vi "Intersect of Line Descriptors.vi"(2 "Line B":T1, 3 "Line A":T1) -> (0 "Intersect":cluster{"X":dbl, "Y":dbl})   [LabVIEW 2012]
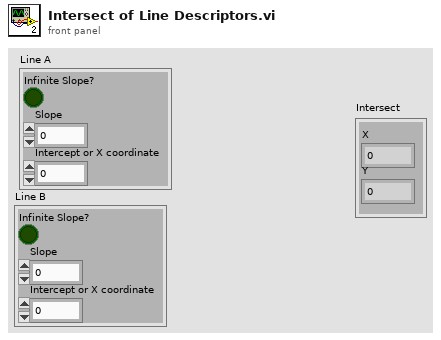
[diagram p1: front panel]
types:
  T1 = cluster{"Infinite Slope?":bool, "Slope":dbl, "Intercept or X coordinate":dbl}
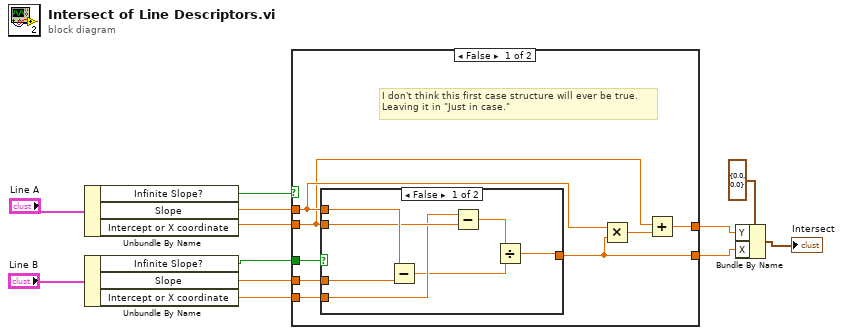
[diagram p0: block diagram]
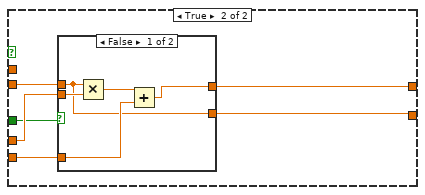
[diagram p3: hidden frame]
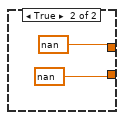
[diagram p4: hidden frame]
diagram:
  n1 = Unbundle By Name("Line A") -> ("Infinite Slope?"=w7:bool, "Slope"=w6:dbl, "Intercept or X coordinate"=w5:dbl)
  n2 = Unbundle By Name("Line B") -> ("Infinite Slope?"=w8:bool, "Slope"=w11:dbl, "Intercept or X coordinate"=w12:dbl)
  n3 = case shown="False" w7 {
    tunnel: w12 -> [w18 w33]
    tunnel: w11 -> [w19 w34]
    tunnel: w8 -> [w20 w30]
    tunnel: w6 -> [w17 _]
    tunnel: w5 -> [w15 w31]
    tunnel: [w14 w29] -> w3
    tunnel: [w13 w32] -> w2
    frame False {
      # "I don't think this first case structure will ever be true.\nLeaving it in \"Just in case.\""
      n4 = case shown="False" w20 {
        tunnel: w17 -> [w27 _]
        tunnel: w15 -> [w25 _]
        tunnel: w19 -> [w26 _]
        tunnel: w18 -> [w24 w28]
        tunnel: [w21 w28] -> w14
        frame False {
          n5 = Subtract(x=w27, y=w26) -> (x-y=w23:dbl)
          n6 = Subtract(x=w24, y=w25) -> (x-y=w22:dbl)
          n7 = Divide(x=w22, y=w23) -> (x/y=w21:dbl)
        }
        frame True {
        }
      }
      n8 = Multiply(x=w17, y=w14) -> (x*y=w16:dbl)
      n9 = Add(x=w15, y=w16) -> (x+y=w13:dbl)
    }
    frame True {
      n10 = case shown="False" w30 {
        tunnel: w34 -> [w39 _]
        tunnel: w33 -> [w37 _]
        tunnel: [w36 nan] -> w32
        tunnel: w31 -> [w35 _]
        tunnel: [w35 nan] -> w29
        frame False {
          n11 = Multiply(x=w35, y=w39) -> (x*y=w38:dbl)
          n12 = Add(x=w38, y=w37) -> (x+y=w36:dbl)
        }
        frame True {
        }
      }
    }
  }
  n13 = Bundle By Name(cluster=cluster{"X":dbl, "Y":dbl} {"X"=0.0, "Y"=0.0} ("Intersect 2"), "Y"=w2, "X"=w3) -> (→"Intersect":cluster{"X":dbl, "Y":dbl})
